vi "XIPIN_Viterbi_Decoder_9_1.vi"   [LabVIEW 2017]
doc: "The Xilinx Viterbi Decoder is fully synchronous, using a single clock. Options include parameterizable constraint length, convolutional codes and traceback length. Various architectures are available including parallel, serial, multi-channel and dual decoding.\n------------------------------------\n<b>Need License</b> : Yes\n<b>Interface</b> : AXI4-Stream"
uses:
  <vilib>/rvi/XilinxIP/XIPIN_XNode/niFpgaXIPIN.xnode
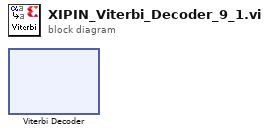
[diagram p0: block diagram]
diagram:
  n1 = xnode ("Viterbi Decoder")() -> ()
